vi "Tests.vi"() -> ()   [LabVIEW 2014]
panel:
  out "CanAcqusiton":bool
  out "FrameIn":u8[](array[numeric])
  out "Frame In":cluster{i32[], "Array":u8[]}(graph)
  out "Frame Nak":cluster{i32[], "Array":u8[]}(graph)
  out "Frame Out":cluster{i32[], "Array":u8[]}(graph)
  out "error out":errorcluster
  in  "Start":bool
  in  "stop":bool
  out "SerialNumber":string
  out "Information":string
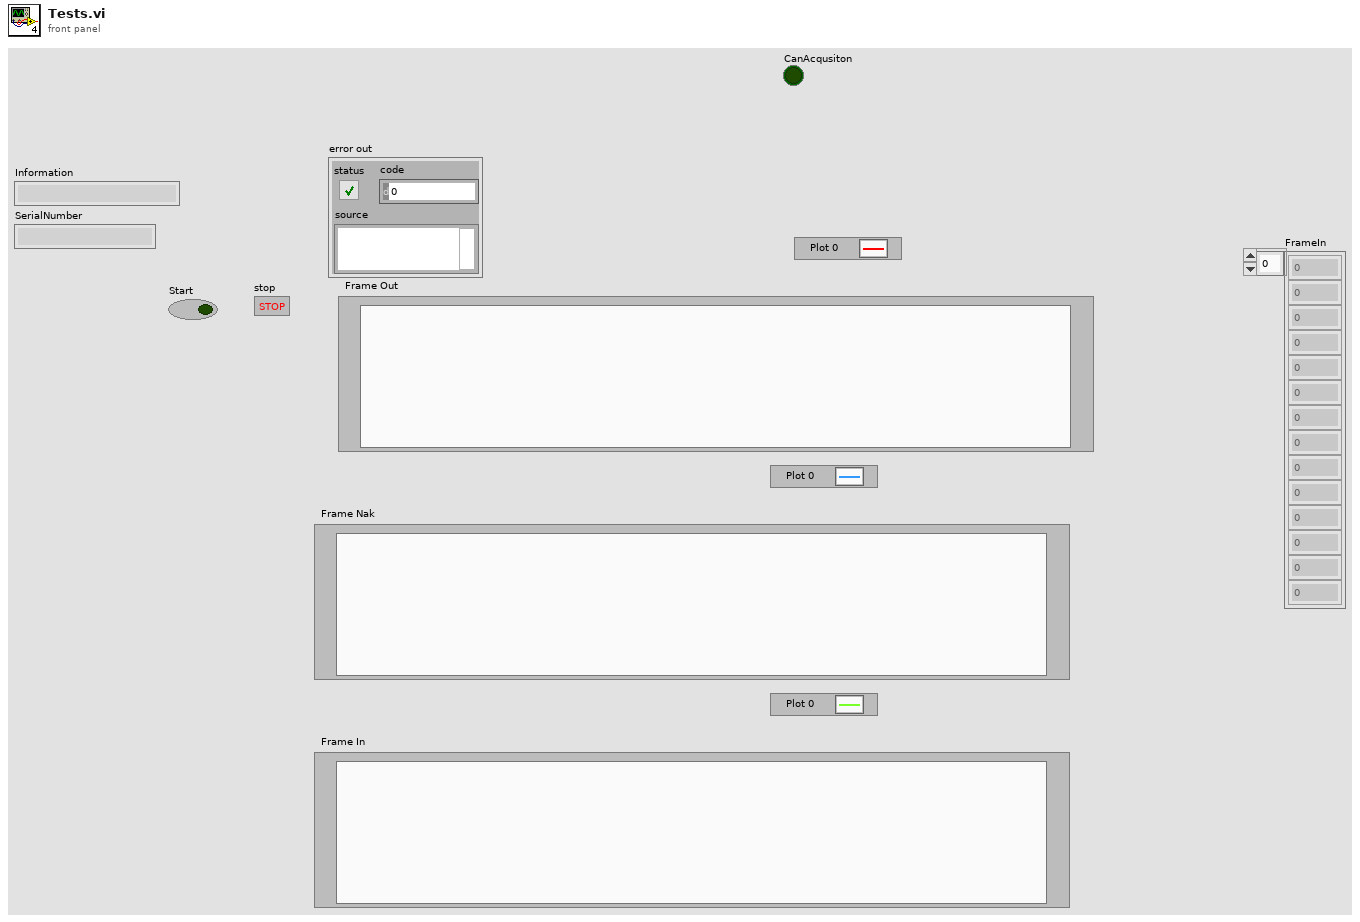
[diagram p1: front panel]
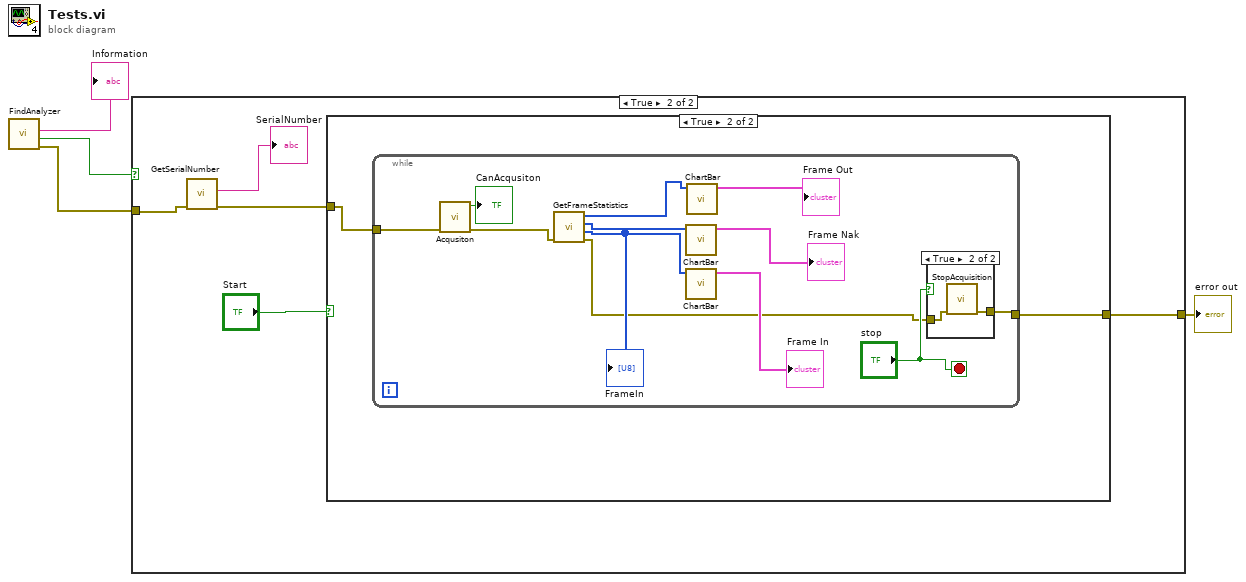
[diagram p0: block diagram]
diagram:
  n1 = call "FindAnalyzer.vi"() -> ("error out"=w2:errorcluster, "IsFound"=w4:bool, "Information"=→"Information":string)  [unwired: 9 in]
  n2 = case shown="True" w4 {
    tunnel: w2 -> [_ w8]
    tunnel: [_ w5] -> w1
    frame False {
    }
    frame True {
      n3 = call "GetSerialNumber.vi"("error in (no error)"=w8) -> ("error out"=w7:errorcluster, "SerialNumber"=→"SerialNumber":string)  [unwired: 9 in]
      n4 = case shown="True" "Start" {
        tunnel: w7 -> [_ w10]
        tunnel: [_ w11] -> w5
        frame False {
        }
        frame True {
          n5 = while {
            tunnel: [w15] -> w11
            tunnel: w10 -> [w14]
            stop <- "stop" stop-if-true
            n6 = call "Acqusiton.vi"("error in (no error)"=w14) -> ("error out"=w13:errorcluster, "CanAcqusiton"=→"CanAcqusiton":bool)  [unwired: 9 in]
            n7 = call "GetFrameStatistics.vi"("error in (no error)"=w13) -> ("error out"=w16:errorcluster, "FrameIn"=w20:u8[], "FrameNak"=w21:u8[], "FrameOut"=w23:u8[])  [unwired: 7 in]
            "FrameIn" <- w20
            n8 = call "ChartBar.vi"("Array"=w21) -> ("XY Graph"=→"Frame Nak":cluster{i32[], "Array":u8[]})  [unwired: 10 in]
            n9 = call "ChartBar.vi"("Array"=w20) -> ("XY Graph"=→"Frame In":cluster{i32[], "Array":u8[]})  [unwired: 10 in]
            n10 = call "ChartBar.vi"("Array"=w23) -> ("XY Graph"=→"Frame Out":cluster{i32[], "Array":u8[]})  [unwired: 10 in]
            n11 = case shown="True" "stop" {
              tunnel: w16 -> [_ w25]
              tunnel: [_ w24] -> w15
              frame False {
              }
              frame True {
                n12 = call "StopAcquisition.vi"("error in (no error)"=w25) -> ("error out"=w24:errorcluster)  [unwired: 9 in, 1 out]
              }
            }
          }
        }
      }
    }
  }
  "error out" <- w1
